vi "UHR-Fleezers Control (host) -Mau_stepping_gamma.vi"(0 "Tab Control":T5(tab)) -> ()   [LabVIEW 2013] (continued)
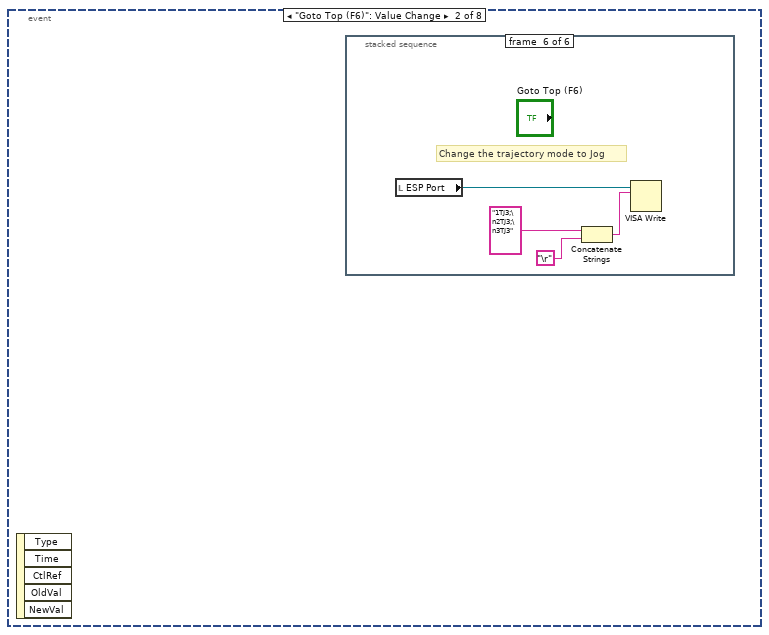
[diagram p4: hidden frame]
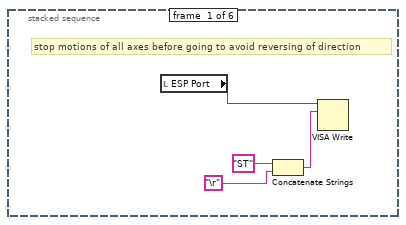
[diagram p5: hidden frame]
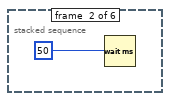
[diagram p6: hidden frame]
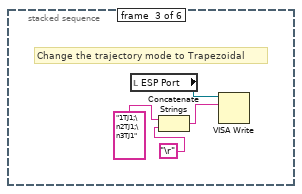
[diagram p7: hidden frame]
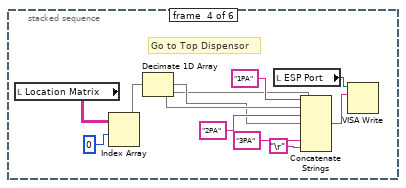
[diagram p8: hidden frame]
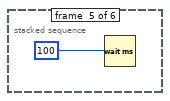
[diagram p9: hidden frame]
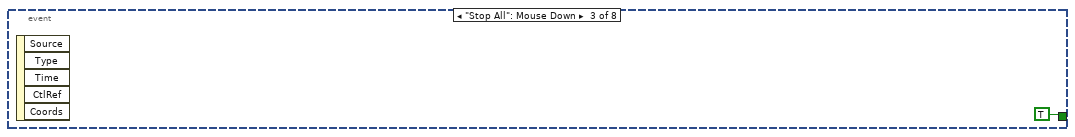
[diagram p10: hidden frame]
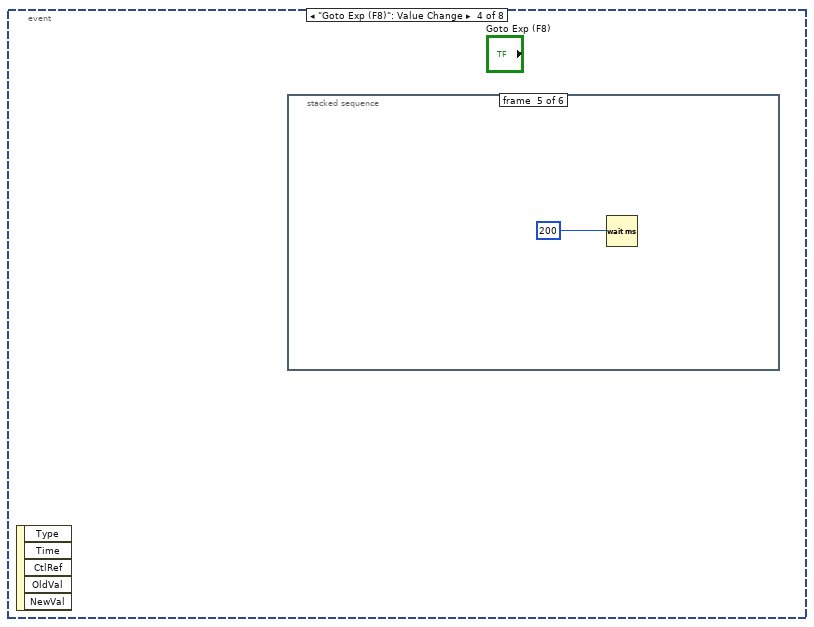
[diagram p11: hidden frame]
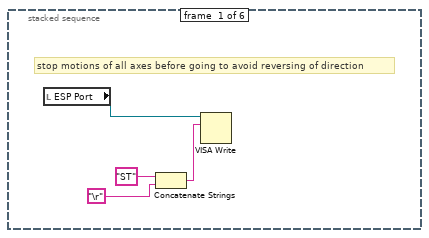
[diagram p12: hidden frame]
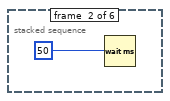
[diagram p13: hidden frame]
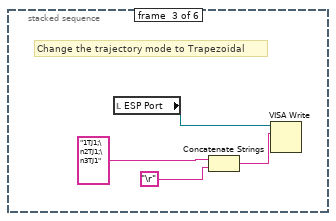
[diagram p14: hidden frame]
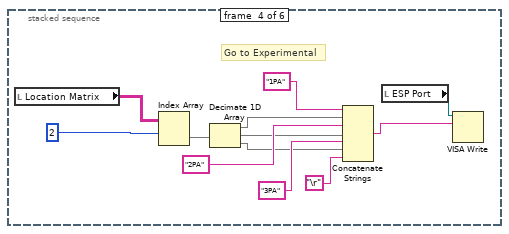
[diagram p15: hidden frame]
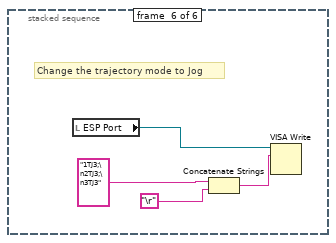
[diagram p16: hidden frame]
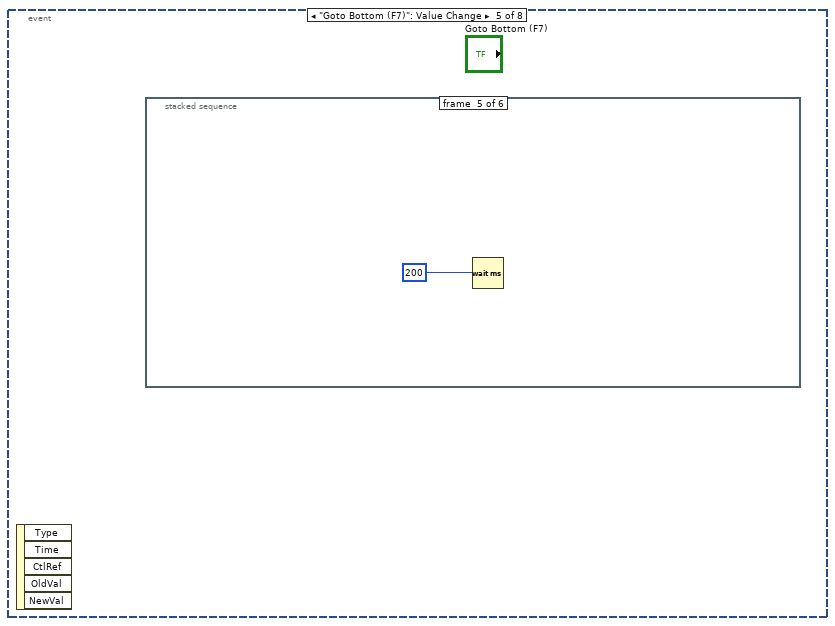
[diagram p17: hidden frame]
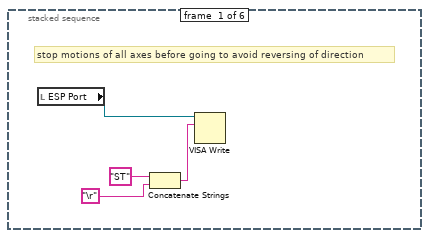
[diagram p18: hidden frame]
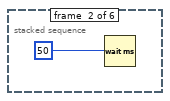
[diagram p19: hidden frame]
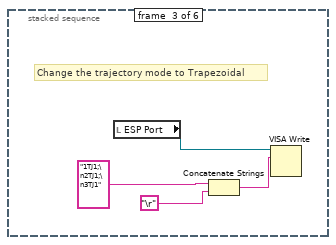
[diagram p20: hidden frame]
                n1984 = To Unsigned Long Integer(number=w3428) -> (unsigned 32bit integer=w3426:u32)
              }
            }
            n1985 = local read "Index"() -> (w3285:dbl)
            n1986 = call "Create new save file.vi"("Insert"="", "Ext"=".dat", "Index In"=w3285) -> ("Path Out"=w3244:path, "Index Out"=w3257:dbl)
            n1987 = local write "Save file name"(w3244) -> ()
            n1988 = local write "Index"(w3257) -> ()
            n1989 = local write "Save index"(w3257) -> ()
            n1990 = Array Size(array=w3268) -> (size(s)=w3269:i32)
            n1991 = Open/Create/Replace File(file path (use dialog)=w3244, operation (0:open)=T23."create", access (0:read/write)=enum16{"read/write", "read-only", "write-only"}."write-only") -> (refnum out=w3282:refnum<file>)  [unwired: 1 in, 4 out]
            n1992 = local write "Saving..."(TRUE ("Saving...")) -> ()
            n1993 = To Double Precision Float(number=w3269) -> (double precision float=w3267:dbl)
            n1994 = String Length(string="Comment (data description)") -> (length=w3265:i32)
            n1995 = To Double Precision Float(number=w3265) -> (double precision float=w3264:dbl)
            n1996 = Deny Access(7:w3282) -> (3:w3281:refnum<file>)  [unwired: 1 in, 2 out]
            n1997 = Build Array (concatenate)(w3267, w3268, w3264) -> (w3266:dbl[])
            n1998 = case "If fluorescence data to be saved" shown="True" w3255 {
              tunnel: w3244 -> [_ w3334]
              tunnel: [refnum<k0> refnum w3314] -> w3256
              frame False {
              }
              frame True {
                w3313 = 0.0
                n1999 = local read "APD Integration Time (s)"() -> (w3319:dbl)
                n2000 = local read "N APD Samp/step"() -> (w3312:dbl)
                n2001 = Path To String(path=w3334) -> (string=w3333:string)
                n2002 = String Length(string=w3333) -> (length=w3332:i32)
                n2003 = Subtract(x=w3332, y=4) -> (x-y=w3330:i32)
                n2004 = String Subset(string=w3333, length (rest)=w3330) -> (substring=w3329:string)  [unwired: 1 out]
                n2005 = Build Array(w3319, w3312, w3313, w3313, w3313, w3313, w3313, w3313) -> (w3316:dbl[])
                n2006 = Concatenate Strings(w3329, "_fl.dat" ("string")) -> (w3327:string)
                n2007 = Array Size(array=w3316) -> (size(s)=w3318:i32)
                n2008 = String To Path(string=w3327) -> (path=w3323:path)
                n2009 = Open/Create/Replace File(file path (use dialog)=w3323, operation (0:open)=T23."create", access (0:read/write)=enum16{"read/write", "read-only", "write-only"}."write-only") -> (refnum out=w3324:refnum<file>)  [unwired: 1 in, 4 out]
                n2010 = Deny Access(7:w3324) -> (3:w3320:refnum<file>)  [unwired: 1 in, 2 out]
                n2011 = To Double Precision Float(number=w3318) -> (double precision float=w3317:dbl)
                n2012 = Build Array (concatenate)(w3317, w3316) -> (w3315:dbl[])
                n2013 = Write to Binary File(file (use dialog)=w3320, data=w3315, 5:FALSE ("prepend array or string size? (T)"), 9:T29."big-endian, network order" ("byte order (0:big-endian, network order)")) -> (refnum out=w3314:refnum<file>)  [unwired: 1 in, 3 out]
              }
            }
            n2014 = case shown="True" w3242 {
              tunnel: w3244 -> [_ w3296]
              tunnel: [refnum<k0> refnum w3295] -> w3243
              frame False {
              }
              frame True {
                w3291 = 0.0 ("element")
                n2015 = Path To String(path=w3296) -> (string=w3310:string)
                n2016 = Build Array(w3291, w3291, w3291, w3291, w3291, w3291, w3291, w3291) -> (w3292:dbl[])
                n2017 = String Length(string=w3310) -> (length=w3309:i32)
                n2018 = Subtract(x=w3309, y=4) -> (x-y=w3307:i32)
                n2019 = Array Size(array=w3292) -> (size(s)=w3294:i32)
                n2020 = String Subset(string=w3310, length (rest)=w3307) -> (substring=w3306:string)  [unwired: 1 out]
                n2021 = To Double Precision Float(number=w3294) -> (double precision float=w3293:dbl)
                n2022 = Concatenate Strings(w3306, "_pos.dat" ("string")) -> (w3304:string)
                n2023 = Build Array (concatenate)(w3293, w3292) -> (w3290:dbl[])
                n2024 = String To Path(string=w3304) -> (path=w3300:path)
                n2025 = Open/Create/Replace File(file path (use dialog)=w3300, operation (0:open)=T23."create", access (0:read/write)=enum16{"read/write", "read-only", "write-only"}."write-only") -> (refnum out=w3301:refnum<file>)  [unwired: 1 in, 4 out]
                n2026 = Deny Access(7:w3301) -> (3:w3297:refnum<file>)  [unwired: 1 in, 2 out]
                n2027 = Write to Binary File(file (use dialog)=w3297, data=w3290, 5:FALSE ("prepend array or string size? (T)"), 9:T29."big-endian, network order" ("byte order (0:big-endian, network order)")) -> (refnum out=w3295:refnum<file>)  [unwired: 1 in, 3 out]
              }
            }
            n2028 = Write to Binary File(file (use dialog)=w3281, data=w3266, 5:w3262, 9:w3260) -> (refnum out=w3263:refnum<file>)  [unwired: 1 in, 3 out]
            n2029 = Write to Binary File(file (use dialog)=w3263, data="Comment (data description)", 5:w3262, 9:w3260) -> (refnum out=w3259:refnum<file>)  [unwired: 1 in, 3 out]
          }
        }
        n2030 = feedback-in #19(w3202) -> ()
        n2031 = feedback-in #20(w3229) -> ()
        n2032 = feedback-in #21(w3201) -> ()
        n2033 = feedback-in #22(w3212) -> ()
        n2034 = feedback-in #23(w3215) -> ()
        n2035 = feedback-in #24(w3228) -> ()
        n2036 = feedback-in #25(w3218) -> ()
      }
      frame #1 {
        n2037 = local read "Saving..."() -> (w3459:bool)
        n2038 = case shown="True" w3459 {
          tunnel: w3463 -> [_ w3473]
          tunnel: w3462 -> [_ w3487]
          tunnel: w3461 -> [_ w3483]
          tunnel: w3460 -> [_ w3482]
          tunnel: w3458 -> [_ w3481]
          tunnel: w3457 -> [_ w3476]
          tunnel: w3456 -> [_ w3475]
          tunnel: w3455 -> [_ w3474]
          tunnel: w3454 -> [_ w3472]
          tunnel: w3453 -> [_ w3470]
          tunnel: w3452 -> [_ w3469]
          tunnel: w3451 -> [_ w3468]
          tunnel: w3450 -> [_ w3467]
          tunnel: w3449 -> [_ w3466]
          tunnel: w3448 -> [_ w3465]
          tunnel: w3447 -> [_ w3464]
          frame False {
          }
          frame True {
            n2039 = Multiply(x=w3473, y=w3472) -> (x*y=→"Time (s)":dbl)
            n2040 = Less Or Equal?(x=w3473, y=w3481) -> (x <= y?=w3485:bool)
            n2041 = Or(x="Stop Saving", y="Abort save 2") -> (x .or. y?=w3477:bool)
            n2042 = Not(x=w3477) -> (.not. x?=w3486:bool)
            n2043 = And(x=w3485, y=w3486) -> (x .and. y?=w3484:bool)
            n2044 = case shown="True" w3484 {
              tunnel: w3487 -> [w3494 w3562]
              tunnel: [0.0 w3565] -> w3480
              tunnel: w3473 -> [_ w3563]
              tunnel: w3481 -> [_ w3564]
              tunnel: w3483 -> [_ w3559]
              tunnel: w3482 -> [_ _]
              tunnel: w3476 -> [w3492 w3552]
              tunnel: w3475 -> [w3491 w3553]
              tunnel: w3474 -> [_ w3551]
              tunnel: w3470 -> [_ w3550]
              tunnel: w3469 -> [_ w3504]
              tunnel: w3468 -> [_ w3543]
              tunnel: w3467 -> [_ w3521]
              tunnel: w3466 -> [w3489 w3502]
              tunnel: w3465 -> [w3490 w3501]
              tunnel: w3464 -> [_ w3498]
              frame False {
                w3488 = FALSE
                n2045 = Close File(refnum=w3494) -> ()  [unwired: 1 in, 2 out]
                n2046 = case shown="True" w3491 {
                  tunnel: w3492 -> [_ w3496]
                  frame False {
                  }
                  frame True {
                    n2047 = Close File(refnum=w3496) -> ()  [unwired: 1 in, 2 out]
                  }
                }
                n2048 = case shown="True" w3489 {
                  tunnel: w3490 -> [_ w3495]
                  frame False {
                  }
                  frame True {
                    n2049 = Close File(refnum=w3495) -> ()  [unwired: 1 in, 2 out]
                  }
                }
                n2050 = local write "Calibrating Trap..."(w3488) -> ()
                n2051 = call <vilib>:"Beep.vi"() -> ()  [unwired: 3 in, 9 out]
                n2052 = local write "Stop Saving"(w3488) -> ()
                n2053 = property on="Raster Scanning..." class="Bool (strict)"("Val(Sgnl)"=w3488) -> ()  [unwired: 2 in, 2 out]
                "Saving..." <- w3488
              }
              frame True {
                n2054 = local read "Calibrating Trap..."() -> (w3554:bool)
                n2055 = case "Write fl. data" shown="True" w3553 {
                  tunnel: w3552 -> [_ w3588]
                  tunnel: w3551 -> [_ w3587]
                  frame False {
                  }
                  frame True {
                    n2056 = Write to Binary File(file (use dialog)=w3588, data=w3587, 5:FALSE ("prepend array or string size? (T)"), 9:T29."big-endian, network order" ("byte order (0:big-endian, network order)")) -> ()  [unwired: 1 in, 4 out]
                  }
                }
                n2057 = Greater?(x="Save ave N", y=1.0) -> (0:w3557:bool)
                n2058 = Not(x=w3554) -> (.not. x?=w3556:bool)
                n2059 = And(x=w3556, y=w3557) -> (x .and. y?=w3499:bool)
                n2060 = case shown="True" w3499 {
                  tunnel: w3498 -> [w3568 w3579]
                  tunnel: [w3568 w3571] -> w3497
                  tunnel: "Save ave N" -> [_ w3572]
                  frame False {
                  }
                  frame True {
                    w3569 = 2 ("dimension size")
                    n2061 = Array Size(array=w3579) -> (size(s)=w3573:i32)
                    n2062 = Divide(x=w3573, y=w3569) -> (x/y=w3577:dbl)
                    n2063 = Reshape Array(w3579, w3577, w3569) -> (w3578:u64[][])
                    n2064 = Transpose 2D Array(2D array=w3578) -> (transposed array=w3576:u64[][])
                    n2065 = for {
                      tunnel: w3576 -> [w3581] mode=indexing
                      tunnel: [w3580] -> w3570 mode=indexing
                      tunnel: w3572 -> [w3582]
                      workers-P: _ -> [_]
                      n2066 = call "downsample 1D array - U64.vi"("Ave N"=w3582, "Array In"=w3581) -> ("Array Out"=w3580:u64[])  [unwired: 1 in]
                    }
                    n2067 = Transpose 2D Array(2D array=w3570) -> (transposed array=w3575:u64[][])
                    n2068 = Divide(x=w3573, y=w3572) -> (x/y=w3574:dbl)
                    n2069 = Reshape Array(w3575, w3574) -> (w3571:u64[])
                  }
                }
                n2070 = case shown="True" w3499 {
                  tunnel: w3559 -> [w3591 w3603]
                  tunnel: [w3591 w3595] -> w3555
                  tunnel: "Save ave N" -> [_ w3596]
                  tunnel: w3550 -> [_ w3594]
                  frame False {
                    # "don't downsample data for trap calibration"
                  }
                  frame True {
                    n2071 = Array Size(array=w3603) -> (size(s)=w3597:i32)
                    n2072 = Array Size(array=w3594) -> (size(s)=w3593:i32)
                    n2073 = Divide(x=w3597, y=w3593) -> (x/y=w3601:dbl)
                    n2074 = Reshape Array(w3603, w3601, w3593) -> (w3602:i16[][])
                    n2075 = Transpose 2D Array(2D array=w3602) -> (transposed array=w3600:i16[][])
                    n2076 = for {
                      tunnel: w3600 -> [w3606] mode=indexing
                      tunnel: [w3605] -> w3592 mode=indexing
                      tunnel: w3596 -> [w3604]
                      workers-P: _ -> [_]
                      n2077 = call "downsample 1D array - I16.vi"("Ave N"=w3604, "Array In"=w3606) -> ("Array Out"=w3605:i16[])  [unwired: 1 out]
                    }
                    n2078 = Transpose 2D Array(2D array=w3592) -> (transposed array=w3599:i16[][])
                    n2079 = Divide(x=w3597, y=w3596) -> (x/y=w3598:dbl)
                    n2080 = Reshape Array(w3599, w3598) -> (w3595:i16[])
                  }
                }
                n2081 = Index Array(array=w3521, index=1) -> (element=w3524:waveform(dbl))
                n2082 = Index Array(array=w3521, index=0) -> (element=w3526:waveform(dbl))
                n2083 = Unbundle By Name(w3524) -> ("Y"=w3528:dbl[])
                n2084 = Unbundle By Name(w3526) -> ("Y"=w3536:dbl[])
                n2085 = case "Write trap pos. data" shown="True" w3502 {
                  tunnel: w3501 -> [_ w3584]
                  tunnel: w3497 -> [_ w3583]
                  frame False {
                  }
                  frame True {
                    n2086 = Write to Binary File(file (use dialog)=w3584, data=w3583, 5:FALSE ("prepend array or string size? (T)"), 9:T29."big-endian, network order" ("byte order (0:big-endian, network order)")) -> ()  [unwired: 1 in, 4 out]
                  }
                }
                n2087 = Write to Binary File(file (use dialog)=w3562, data=w3555, 5:FALSE ("prepend array or string size? (T)"), 9:T29."big-endian, network order" ("byte order (0:big-endian, network order)")) -> ()  [unwired: 1 in, 4 out]
                n2088 = feedback #26(w3528) -> (w3530:dbl[])
                n2089 = Build Array (concatenate)(w3530, w3528) -> (w3529:dbl[])
                n2090 = Select(t=w3528, s=w3504, f=w3529) -> (s? t:f=w3514:dbl[])
                n2091 = feedback-in #26(w3514) -> ()
                n2092 = feedback #27(w3536) -> (w3549:dbl[])
                n2093 = Build Array (concatenate)(w3549, w3536) -> (w3548:dbl[])
                n2094 = Select(t=w3536, s=w3504, f=w3548) -> (s? t:f=w3523:dbl[])
                n2095 = feedback-in #27(w3523) -> ()
                n2096 = Divide(x=w3563, y=w3564) -> (x/y=w3566:dbl)
                n2097 = Multiply(x=w3566, y=100.0) -> (x*y=w3565:dbl)
                n2098 = Build Array(w3523, w3514) -> (→"Saved APD":dbl[][])
                n2099 = Array Size(array=w3523) -> (size(s)=w3541:i32)
                n2100 = Unbundle By Name(w3543) -> ("Y"=w3547:dbl[])
                n2101 = Subtract(x=w3541, y="N pts to average") -> (x-y=w3517:i32)
                n2102 = Multiply(x="N pts to average", y=u16 2) -> (x*y=w3518:u16)
                n2103 = Subtract(x=w3541, y=w3518) -> (x-y=w3516:i32)
                n2104 = feedback #28(w3547) -> (w3546:dbl[])
                n2105 = Build Array (concatenate)(w3546, w3547) -> (w3545:dbl[])
                n2106 = Select(t=w3547, s=w3504, f=w3545) -> (s? t:f=w3544:dbl[])
                "Trap Delta Graph" <- w3544
                n2107 = feedback-in #28(w3544) -> ()
                n2108 = Array Subset(array=w3523, index=w3517, length="N pts to average") -> (w3540:dbl[])
                n2109 = Array Subset(array=w3523, index=w3516, length="N pts to average") -> (w3539:dbl[])
                n2110 = Array Subset(array=w3514, index=w3517, length="N pts to average") -> (w3520:dbl[])
                n2111 = Array Subset(array=w3514, index=w3516, length="N pts to average") -> (w3519:dbl[])
                n2112 = call-poly <vilib>:"Mean.vi"("X"=w3540) -> ("mean"=w3538:dbl)  [unwired: 1 out]
                n2113 = call-poly <vilib>:"Mean.vi"("X"=w3520) -> ("mean"=w3513:dbl)  [unwired: 1 out]
                n2114 = call-poly <vilib>:"Mean.vi"("X"=w3539) -> ("mean"=w3537:dbl)  [unwired: 1 out]
                n2115 = call-poly <vilib>:"Mean.vi"("X"=w3519) -> ("mean"=w3512:dbl)  [unwired: 1 out]
                n2116 = Subtract(x=w3513, y=w3512) -> (x-y=w3503:dbl)
                "Delta Fl. 2" <- w3503
                n2117 = Subtract(x=w3538, y=w3537) -> (x-y=w3535:dbl)
                "Delta Fl. 1" <- w3535
                n2118 = Initialize Array(w3535, 1 ("dimension size")) -> (w3532:dbl[])
                n2119 = Initialize Array(w3503, 1 ("dimension size")) -> (w3509:dbl[])
                n2120 = feedback #29(w3532) -> (w3533:dbl[])
                n2121 = Build Array (concatenate)(w3533, w3532) -> (w3531:dbl[])
                n2122 = feedback #30(w3509) -> (w3510:dbl[])
                n2123 = Build Array (concatenate)(w3510, w3509) -> (w3508:dbl[])
                n2124 = Select(t=w3532, s=w3504, f=w3531) -> (s? t:f=w3507:dbl[])
                n2125 = feedback-in #29(w3507) -> ()
                n2126 = Select(t=w3509, s=w3504, f=w3508) -> (s? t:f=w3506:dbl[])
                n2127 = feedback-in #30(w3506) -> ()
                n2128 = Build Array(w3507, w3506) -> (→"Save APD Deriv":dbl[][])
              }
            }
            "Progress" <- w3480
            "Progress 2" <- w3480
          }
        }
      }
    }
    n2129 = Bundle By Name(cluster=w2224, "Green FB Ch 0"=w2223, "Green FB Ch 1"=w2222) -> (w2202:T48)
    "Green FB Signals (V)" <- w2202
    n2130 = Unbundle By Name(w2202) -> ("Green FB Ch 2"=→"Green FB Plot":dbl)
    n2131 = local read "wait to reset values"() -> (w2294:bool)
    n2132 = Not(x=w2291) -> (.not. x?=w2295:bool)
    n2133 = And(x=w2295, y=w2294) -> (x .and. y?=w2296:bool)
    n2134 = case "Part of MCL raster scanning: returns to initial positions after scan done" shown="False" w2296 {
      tunnel: w2299 -> [w3032 w3039]
      tunnel: [w3032 w3038] -> w2298
      tunnel: w2293 -> [w3031 w3037]
      tunnel: [w3031 w3036] -> w2292
      frame False {
      }
      frame True {
        w3047 = 10.0 ("y")
        w3046 = 32767.0 ("y")
        # "to return scan values\nafter a synchronous \nAOM scan"
        n2135 = local read "AO2"() -> (w3040:dbl)
        n2136 = local read "AO1"() -> (w3041:dbl)
        n2137 = local write "wait to reset values"(FALSE ("wait to reset values")) -> ()
        n2138 = Multiply(x=w3041, y=w3046) -> (x*y=w3043:dbl)
        n2139 = Multiply(x=w3040, y=w3046) -> (x*y=w3045:dbl)
        n2140 = Divide(x=w3043, y=w3047) -> (x/y=w3042:dbl)
        n2141 = Divide(x=w3045, y=w3047) -> (x/y=w3044:dbl)
        n2142 = To Word Integer(number=w3042) -> (16bit integer=w3048:i16)
        n2143 = To Word Integer(number=w3044) -> (16bit integer=w3049:i16)
        n2144 = local read "Total Counts (ticks)"() -> (w3033:u32)
        n2145 = xnode "Read/Write Control"("FPGA VI Reference In"=w3039, "error in"=w3037, "AO1"=w3048, "AO2"=w3049, "MCL count"=w3033) -> ("FPGA VI Reference Out"=w3038:T19, "error out"=w3036:errorcluster)
        n2146 = local read "Scan Range (V)\n(of steps)"() -> (w3034:dbl)
        n2147 = property on="Scan Range (V)\n(of steps)" class="DigNum (strict)"("Val(Sgnl)"=w3034) -> ()  [unwired: 2 in, 2 out]
      }
    }
    n2148 = node-c288() -> ()  [unwired: 2 out]
  }
  n2149 = node-c288(3 ("Processor")) -> (w74:T24)  [unwired: 3 out]
  n2150 = timed-loop "Oscillate AOD (debugging)" {
    tunnel: w24 -> [w3608]
    tunnel: [w3607] -> w36
    timing: w74 -> [_]
    timing-out: [_] -> w73
    stop <- w3607 stop-if-true
    n2151 = node-c288() -> ()  [unwired: 2 out]
    n2152 = event shown="[0] \"Oscillate Set 2\", \"Fish for Tether\": Value Change" {
      selector: _ -> [_ _ _]
      dyn-events: _ -> [_ _ _]
      timeout: _ -> [_ _ _]
      tunnel: w3608 -> [w3615 _ _]
      tunnel: [FALSE ("Stop All") _ w3890] -> w3607
      event "Oscillate Set 2", "Fish for Tether": Value Change {
        n2153 = event-data() -> ()  [unwired: 6 out]
        n2154 = local read "Oscillate Set 2"() -> (w3614:bool)
        n2155 = Or(x=w3614, y="Fish for Tether") -> (x .or. y?=w3612:bool)
        n2156 = case shown="True" w3612 {
          tunnel: w3615 -> [_ w3618]
          tunnel: "Fish for Tether" -> [_ w3617]
          frame False {
          }
          frame True {
            n2157 = case shown="True" w3617 {
              frame False {
              }
              frame True {
                n2158 = local write "Scan axis 2"(TRUE) -> ()
                n2159 = local write "Tether"(FALSE ("Tether")) -> ()
              }
            }
            n2160 = node-c288("Period") -> (w3620:T24)  [unwired: 3 out]
            n2161 = timed-loop "Oscillate AOD" {
              timing: w3620 -> [_]
              timing-out: [_] -> w3619
              tunnel: w3618 -> [w3630]
              tunnel: w3617 -> [w3629]
              i -> [w3632]
              stop <- w3628 stop-if-true
              n2162 = node-c288() -> (w3631:i64)  [unwired: 1 out]
              n2163 = flat-sequence {
                tunnel: w3632 -> [w3658]
                tunnel: w3631 -> [w3657]
                tunnel: w3630 -> [w3641]
                tunnel: w3629 -> [w3643]
                tunnel: [w3643] -> w3627
                tunnel: [w3642] -> w3626
                tunnel: [w3640] -> w3625
                tunnel: [w3637] -> w3623
                tunnel: w3627 -> [w3701]
                tunnel: w3626 -> [w3699]
                tunnel: w3625 -> [w3698]
                tunnel: [w3697] -> w3624
                tunnel: w3623 -> [w3696]
                tunnel: [w3765] -> w3628
                tunnel: w3624 -> [w3763]
                frame #0 {
                  n2164 = Divide(x=w3657, y=i64 1000) -> (x/y=w3652:dbl)
                  n2165 = Multiply(x=w3652, y=w3658) -> (x*y=w3654:dbl)
                  n2166 = Multiply(x="Osc. freq. (Hz)", y=6.283185307179586) -> (x*y=w3655:dbl)
                  n2167 = Multiply(x=w3655, y=w3654) -> (x*y=w3639:dbl)
                  n2168 = local read "BD 1 Frequency 2 (MHz)"() -> (w3636:dbl)
                  n2169 = local read "BD 1 Frequency 1 (MHz)"() -> (w3633:dbl)
                  n2170 = case shown="True" w3643 {
                    tunnel: w3639 -> [w3664 w3679]
                    tunnel: w3636 -> [_ w3689]
                    tunnel: [w3661 w3673] -> w3644
                    tunnel: [FALSE w3682] -> w3640
                    tunnel: [0.0 w3675] -> w3637
                    tunnel: w3633 -> [_ w3674]
                    frame False {
                      n2171 = Sine(x=w3664) -> (sin(x)=w3662:dbl)
                      n2172 = Multiply(x=w3662, y="Osc. amp. (MHz)") -> (x*y=w3661:dbl)
                    }
                    frame True {
                      n2173 = Cosine(x=w3679) -> (cos(x)=w3672:dbl)
                      n2174 = Subtract(x=w3689, y=w3674) -> (x-y=w3688:dbl)
                      n2175 = Equal?(x=-1, y=w3672) -> (x = y?=w3670:bool)
                      n2176 = Decrement(x=w3672) -> (x-1=w3691:dbl)
                      n2177 = Subtract(x=w3688, y="Closest Delta (MHz)") -> (x-y=w3685:dbl)
                      n2178 = Select(t="Pause at Closest Delta (s)", s=w3670, f=0) -> (s? t:f=w3668:dbl)
                      n2179 = Divide(x=w3691, y=2.0) -> (x/y=w3686:dbl)
                      n2180 = Multiply(x=1000, y=w3668) -> (x*y=w3666:dbl)
                      n2181 = Multiply(x=w3686, y=w3685) -> (x*y=w3673:dbl)
                      n2182 = local read "Vec Mean of T1 T2"() -> (w3681:dbl[])
                      n2183 = Wait (ms)(milliseconds to wait=w3666) -> ()  [unwired: 1 out]
                      n2184 = Greater?(x=w3681, y="Stop F (pN)") -> (0:w3683:bool[])
                      n2185 = Or Array Elements(Boolean array=w3683) -> (logical OR=w3682:bool)
                      n2186 = Divide(x=w3679, y=6.283185307179586) -> (x/y=w3678:dbl)
                      n2187 = Round Toward +Infinity(x=w3678) -> (ceil(x): smallest int >= x=w3675:dbl)
                      "Attempts" <- w3675
                      n2188 = Greater?(x=w3675, y="Attempt Limit") -> (0:w3677:bool)
                      n2189 = case shown="True" w3677 {
                        frame False {
                        }
                        frame True {
                          n2190 = local write "Fish for Tether"(FALSE ("Fish for Tether")) -> ()
                          n2191 = call <vilib>:"Beep.vi"() -> ()  [unwired: 3 in, 9 out]
                          n2192 = local read "Messages"() -> (w3693:string)
                          n2193 = call "Update messages.vi"("Message to add"="Tether fishing timeout." ("Messages"), "Old message string"=w3693) -> ("New message string"=→"Messages":string)
                        }
                      }
                    }
                  }
                  n2194 = local read "Y RF Frequency Limits (MHz)"() -> (w3645:T16)
                  n2195 = local read "X RF Frequency Limits (MHz)"() -> (w3646:T16)
                  n2196 = local read "BD 1 Frequency 3 (MHz)"() -> (w3651:dbl)
                  n2197 = local read "BD 2 Frequency 2 (MHz)"() -> (w3635:dbl)
                  n2198 = Select(t=w3636, s="Scan axis 2", f=w3635) -> (s? t:f=w3647:dbl)
                  n2199 = Add(x=w3644, y=w3647) -> (x+y=w3642:dbl)
                  n2200 = Select(t=w3642, s="Scan axis 2", f=w3636) -> (s? t:f=w3634:dbl)
                  n2201 = Select(t=w3635, s="Scan axis 2", f=w3642) -> (s? t:f=w3649:dbl)
                  n2202 = local read "BD 2 Frequency 3 (MHz)"() -> (w3650:dbl)
                  n2203 = call "set RF board frequency - interlace.vi"("Board 2 Frequency Limits"=w3645, "Board 1 Frequency Limits"=w3646, "FPGA VI Reference In"=w3641, "Board 2 Frequency 3 (MHz)"=w3650, "Board 1 Frequency 3 (MHz)"=w3651, "Board 2 Frequency 2 (MHz)"=w3635, "Board 2 Frequency 1 (MHz)"=w3649, "Board 1 Frequency 2 (MHz)"=w3634, "Board 1 Frequency 1  (MHz)"=w3633) -> ()  [unwired: 1 in, 2 out]
                }
                frame #1 {
                  n2204 = And(x=w3701, y=w3698) -> (x .and. y?=w3700:bool)
                  n2205 = case "Only if were fishing and now formed tether" shown="True" w3700 {
                    tunnel: w3699 -> [w3703 w3715]
                    tunnel: [w3702 w3714] -> w3697
                    tunnel: w3696 -> [_ w3710]
                    frame False {
                      n2206 = local read "Fish for Tether"() -> (w3702:bool)
                      n2207 = case shown="True" w3702 {
                        tunnel: w3703 -> [_ _]
                        frame False {
                        }
                        frame True {
                        }
                      }
                    }
                    frame True {
                      w3714 = FALSE ("Fish for Tether")
                      n2208 = call <vilib>:"Beep.vi"() -> ()  [unwired: 3 in, 9 out]
                      n2209 = Number To Decimal String(number=w3710, width (-)=i16 1) -> (decimal integer string=w3708:string)
                      n2210 = case shown="\"2\", \"3\", \"4\", \"5\", \"6\"" "Then..." {
                        selector: "Then..." -> [_ w3718]
                        tunnel: w3715 -> [w3717 _]
                        frame "1", Default {
                          # "do nothing"
                          n2211 = property on="BD 1 Frequency 1 (MHz)" class="DigNum (strict)"("Val(Sgnl)"=w3717) -> ()  [unwired: 2 in, 2 out]
                        }
                        frame "2", "3", "4", "5", "6" {
                          n2212 = flat-sequence {
                            tunnel: w3718 -> [w3720]
                            frame #0 {
                              n2213 = property on="Trap Delta (MHz)" class="DigNum (strict)"("Val(Sgnl)"="Move to Delta 1 (MHz)") -> ()  [unwired: 2 in, 2 out]
                            }
                            frame #1 {
                              n2214 = case shown="\"5\", \"6\"" w3720 {
                                selector: w3720 -> [w3723 w3733 _]
                                frame "3", "4" {
                                n2215 = flat-sequence {
                                tunnel: w3723 -> [w3724]
                                tunnel: [w3724] -> w3721
                                tunnel: [w3726] -> w3722
                                tunnel: w3721 -> [w3726]
                                tunnel: w3722 -> [w3730]
                                frame #0 {
                                n2216 = property on="Green Laser ON/Interlacing" class="Bool (strict)"("Val(Sgnl)"=TRUE ("Value (Signaling)")) -> ()  [unwired: 2 in, 2 out]
                                }
                                frame #1 {
                                n2217 = Multiply(x="Wait Before Save (s)", y=u32 1000 ("x")) -> (x*y=w3728:u32)
                                n2218 = Wait (ms)(milliseconds to wait=w3728) -> ()  [unwired: 1 out]
                                }
                                frame #2 {
                                n2219 = property on="Start Saving" class="Bool (strict)"("Value"=TRUE ("Start Saving")) -> ()  [unwired: 2 in, 2 out]
                                n2220 = case shown="Default" w3730 {
                                frame Default {
                                }
                                frame "4" {
                                n2221 = property on="Fl. Triggered..." class="Bool (strict)"("Val(Sgnl)"=TRUE ("Value (Signaling)")) -> ()  [unwired: 2 in, 2 out]
                                }
                                }
                                }
                                }
                                }
                                frame "5", "6" {
                                n2222 = stacked-sequence {
                                tunnel: w3733 -> [_ _ _ _ _ _ _ _ w3750 _ _]
                                frame #0 {
                                n2223 = Replace Array Subset(array=u32[] [0] ("Index Values"), new element="Raster Set Upon Tether", index=0) -> (w3734:u32[])
                                n2224 = property on="Saved AOD Raster Scan Parameter Sets" class="Arr (strict)"("Index Values"=w3734) -> ()  [unwired: 2 in, 2 out]
                                }
                                frame #1 {
                                n2225 = Wait (ms)(milliseconds to wait=u32 500) -> ()  [unwired: 1 out]
                                }
                                frame #2 {
                                n2226 = property on="Load parameters" class="Bool (strict)"("Val(Sgnl)"=TRUE ("Value (Signaling)")) -> ()  [unwired: 2 in, 2 out]
                                }
                                frame #3 {
                                n2227 = Wait (ms)(milliseconds to wait=u32 500) -> ()  [unwired: 1 out]
                                }
                                frame #4 {
                                n2228 = property on="Trap Raster Scan" class="Bool (strict)"("Val(Sgnl)"=TRUE ("Value (Signaling)")) -> ()  [unwired: 2 in, 2 out]
                                }
                                frame #5 {
                                n2229 = Wait (ms)(milliseconds to wait=u32 2000) -> ()  [unwired: 1 out]
                                }
                                frame #6 {
                                n2230 = while {
                                stop <- w3745 stop-if-true
                                n2231 = local read "Raster Scanning..."() -> (w3744:bool)
                                n2232 = local read "Saving..."() -> (w3747:bool)
                                n2233 = Wait (ms)(milliseconds to wait=u32 100) -> ()  [unwired: 1 out]
                                n2234 = Not(x=w3747) -> (.not. x?=w3746:bool)
                                n2235 = Not(x=w3744) -> (.not. x?=w3743:bool)
                                n2236 = And(x=w3746, y=w3743) -> (x .and. y?=w3745:bool)
                                }
                                }
                                frame #7 {
                                n2237 = property on="Trap Delta (MHz)" class="DigNum (strict)"("Val(Sgnl)"="Move to Delta 2 (MHz)") -> ()  [unwired: 2 in, 2 out]
                                }
                                frame #8 {
                                n2238 = local read "Tether"() -> (w3751:bool)
                                n2239 = case shown="True" w3751 {
                                tunnel: w3750 -> [_ w3752]
                                frame False {
                                }
                                frame True {
                                n2240 = flat-sequence {
                                tunnel: w3752 -> [w3754]
                                frame #0 {
                                n2241 = Wait (ms)(milliseconds to wait=u32 500) -> ()  [unwired: 1 out]
                                }
                                frame #1 {
                                n2242 = case shown="\"6\"" w3754 {
                                frame Default {
                                }
                                frame "6" {
                                n2243 = property on="Green Laser ON/Interlacing" class="Bool (strict)"("Val(Sgnl)"=TRUE ("Green Laser ON/Interlacing")) -> ()  [unwired: 2 in, 2 out]
                                }
                                }
                                }
                                frame #2 {
                                n2244 = Wait (ms)(milliseconds to wait=u32 500) -> ()  [unwired: 1 out]
                                }
                                frame #3 {
                                n2245 = local write "Start Saving"("Save at end (5, 6)") -> ()
                                }
                                }
                                }
                                }
                                }
                                frame #9 {
                                n2246 = local read "Bead Sep. Int. Time (s)"() -> (w3760:dbl)
                                n2247 = Multiply(x=w3760, y=1000.0) -> (x*y=w3759:dbl)
                                n2248 = Wait (ms)(milliseconds to wait=w3759) -> ()  [unwired: 1 out]
                                }
                                frame #10 {
                                n2249 = property on="Rescale on Mean" class="Bool (strict)"("Val(Sgnl)"=TRUE ("Value (Signaling)")) -> ()  [unwired: 2 in, 2 out]
                                }
                                }
                                }
                                frame "2", Default {
                                }
                              }
                            }
                          }
                        }
                      }
                      n2250 = Concatenate Strings("Formed tether in ", w3708, " attempt(s)." ("string")) -> (w3705:string)
                      n2251 = local read "Messages"() -> (w3712:string)
                      n2252 = local write "Fish for Tether"(w3714) -> ()
                      n2253 = call "Update messages.vi"("Message to add"=w3705, "Old message string"=w3712) -> ("New message string"=w3711:string)
                      n2254 = local write "Messages"(w3711) -> ()
                      n2255 = Get Date/Time In Seconds() -> (seconds since 1Jan1904=→"Time tether formed":timestamp)
                      "Tether" <- "Tether Alarm?"
                    }
                  }
                }
                frame #2 {
                  n2256 = local read "Oscillate Set 2"() -> (w3764:bool)
                  n2257 = local read "Stop All"() -> (w3766:bool)
                  n2258 = Not Or(1:w3763, 2:w3764) -> (0:w3762:bool)
                  n2259 = Compound Arithmetic op=OR(w3766, w3762) -> (w3765:bool)
                }
              }
              n2260 = node-c288() -> ()  [unwired: 2 out]
            }
            n2261 = node-c288(w3619) -> ()  [unwired: 1 out]
          }
        }
      }
      event "Fl. Triggered...": Value Change {
        n2262 = event-data() -> ()  [unwired: 7 out]
        n2263 = case shown="True" "Fl. Triggered..." {
          frame False {
          }
          frame True {
            n2264 = node-c288() -> (w3778:T24)  [unwired: 4 out]
            n2265 = timed-loop {
              timing: w3778 -> [_]
              timing-out: [_] -> w3777
              tunnel: "Action" -> [w3782]
              shift-right: [w3779] -> _
              shift-left: u8 255 -> [w3781]
              stop <- w3783 stop-if-true
              n2266 = node-c288() -> ()  [unwired: 2 out]
              n2267 = flat-sequence {
                tunnel: w3782 -> [w3795]
                tunnel: w3781 -> [w3792]
                tunnel: [w3791] -> w3780
                tunnel: [w3881] -> w3783
                tunnel: w3780 -> [w3880]
                tunnel: [w3880] -> w3779
                frame #0 {
                  n2268 = local read "Delta Fl. 2"() -> (w3786:dbl)
                  n2269 = local read "Delta Fl. 1"() -> (w3787:dbl)
                  n2270 = Select(t=w3787, s="APD to Watch", f=w3786) -> (s? t:f=w3785:dbl)
                  n2271 = Multiply(x="Fl. Delta Thresh. (kHz)", y=1000.0) -> (x*y=w3794:dbl)
                  n2272 = Greater?(x=w3785, y=w3794) -> (0:w3789:bool)
                  n2273 = Or(x="Force Yank", y=w3789) -> (x .or. y?=w3790:bool)
                  n2274 = case shown="True" w3790 {
                    tunnel: w3795 -> [_ w3805]
                    tunnel: w3792 -> [w3797 w3801]
                    tunnel: [w3797 w3798] -> w3791
                    frame False {
                    }
                    frame True {
                      n2275 = flat-sequence {
                        tunnel: w3802 -> [w3811]
                        tunnel: [w3811] -> w3806
                        tunnel: w3805 -> [w3810]
                        tunnel: [w3810] -> w3804
                        tunnel: [w3809] -> w3803
                        tunnel: w3801 -> [w3808]
                        tunnel: [w3807] -> w3800
                        tunnel: w3806 -> [w3836]
                        tunnel: w3804 -> [w3835]
                        tunnel: w3803 -> [w3834]
                        tunnel: w3800 -> [w3833]
                        tunnel: [w3833] -> w3799
                        tunnel: w3799 -> [w3878]
                        tunnel: [w3878] -> w3798
                        frame #0 {
                          n2276 = call <vilib>:"Beep.vi"() -> ()  [unwired: 3 in, 9 out]
                          n2277 = local write "Waiting"(FALSE ("Waiting")) -> ()
                          n2278 = Increment(x=w3808) -> (x+1=w3807:u8)
                          n2279 = case shown="\"Yank\"" w3810 {
                            tunnel: w3807 -> [_ _ w3817]
                            frame "Image" {
                              n2280 = property on="Confocal Image" class="Bool (strict)"("Val(Sgnl)"=TRUE ("Value (Signaling)")) -> ()  [unwired: 2 in, 2 out]
                            }
                            frame "Alarm", Default {
                            }
                            frame "Yank" {
                              n2281 = flat-sequence {
                                tunnel: w3817 -> [w3820]
                                tunnel: [w3819] -> w3816
                                tunnel: ["N Array El"] -> w3815
                                tunnel: w3816 -> [w3830]
                                tunnel: w3815 -> [w3826]
                                frame #0 {
                                n2282 = Multiply(x="Yank Delay (s)", y=1000.0) -> (x*y=w3823:dbl)
                                n2283 = Quotient & Remainder(x=w3820, y="N Array El") -> (x-y*floor(x/y)=w3819:u8)  [unwired: 1 out]
                                n2284 = Wait (ms)(milliseconds to wait=w3823) -> ()  [unwired: 1 out]
                                }
                                frame #1 {
                                n2285 = Random Number (0-1)() -> (number: 0 to 1=w3827:dbl)
                                n2286 = Multiply(x=w3826, y=w3827) -> (x*y=w3825:dbl)
                                n2287 = Round Toward -Infinity(1:w3825) -> (0:w3824:dbl)
                                n2288 = Select(t=w3824, s="Random Choice", f=w3830) -> (s? t:f=w3828:dbl)
                                n2289 = Index Array(array="Yank to Delta Array (MHz)", index=w3828) -> (element=w3831:dbl)
                                n2290 = property on="Trap Delta (MHz)" class="DigNum (strict)"("Val(Sgnl)"=w3831) -> ()  [unwired: 2 in, 2 out]
                                }
                              }
                            }
                          }
                          n2291 = local read "Time (s)"() -> (w3809:dbl)
                          "Fl. High" <- TRUE ("Yanking")
                        }
                        frame #1 {
                          n2292 = node-c288() -> (w3838:T24)  [unwired: 4 out]
                          n2293 = timed-loop {
                            timing: w3838 -> [_]
                            timing-out: [_] -> w3837
                            tunnel: w3836 -> [w3854]
                            tunnel: w3835 -> [w3852]
                            tunnel: w3834 -> [w3851]
                            stop <- w3853 stop-if-true
                            n2294 = node-c288() -> ()  [unwired: 2 out]
                            n2295 = local read "Fl. Delta Thresh. (kHz)"() -> (w3846:dbl)
                            n2296 = local read "Fl. Triggered..."() -> (w3855:bool)
                            n2297 = local read "Delta Fl. 1"() -> (w3842:dbl)
                            n2298 = local read "Delta Fl. 2"() -> (w3840:dbl)
                            n2299 = local read "Stop All"() -> (w3849:bool)
                            n2300 = local read "APD to Watch"() -> (w3841:bool)
                            n2301 = Select(t=w3842, s=w3841, f=w3840) -> (s? t:f=w3839:dbl)
                            n2302 = Not(x=w3855) -> (.not. x?=w3850:bool)
                            n2303 = Multiply(x=w3846, y=1000.0) -> (x*y=w3845:dbl)
                            n2304 = Negate(x=w3845) -> (-x=w3844:dbl)
                            n2305 = Less?(x=w3839, y=w3844) -> (x < y?=w3848:bool)
                            n2306 = Compound Arithmetic op=OR(w3848, w3849, w3850, "Force Reset") -> (w3853:bool)
                            n2307 = case shown="True" w3853 {
                              tunnel: w3854 -> [_ w3866]
                              tunnel: w3852 -> [_ w3865]
                              tunnel: w3851 -> [_ w3863]
                              frame False {
                              }
                              frame True {
                                n2308 = case shown="\"Yank\"" w3865 {
                                tunnel: w3866 -> [_ w3867]
                                frame "Image", Default {
                                }
                                frame "Yank" {
                                n2309 = flat-sequence {
                                tunnel: [w3872] -> w3868
                                tunnel: w3867 -> [w3872]
                                tunnel: w3868 -> [w3873]
                                frame #0 {
                                n2310 = local read "Yank Delay (s)"() -> (w3871:dbl)
                                n2311 = Multiply(x=w3871, y=1000.0) -> (x*y=w3869:dbl)
                                n2312 = Wait (ms)(milliseconds to wait=w3869) -> ()  [unwired: 1 out]
                                }
                                frame #1 {
                                n2313 = property on="Trap Delta (MHz)" class="DigNum (strict)"("Val(Sgnl)"=w3873) -> ()  [unwired: 2 in, 2 out]
                                }
                                }
                                }
                                }
                                n2314 = local read "Time (s)"() -> (w3864:dbl)
                                n2315 = Subtract(x=w3864, y=w3863) -> (x-y=w3860:dbl)
                                "Duration (s)" <- w3860
                                n2316 = Number To Decimal String(number=w3860, width (-)=i16 0) -> (decimal integer string=w3858:string)
                                n2317 = Concatenate Strings(w3858, " s fluorescence event." ("string")) -> (w3856:string)
                                n2318 = local read "Messages"() -> (w3862:string)
                                n2319 = call "Update messages.vi"("Message to add"=w3856, "Old message string"=w3862) -> ("New message string"=w3861:string)
                                n2320 = call <vilib>:"Beep.vi"() -> ()  [unwired: 3 in, 9 out]
                                n2321 = local write "Messages"(w3861) -> ()
                              }
                            }
                            n2322 = node-c288() -> ()  [unwired: 2 out]
                          }
                          n2323 = node-c288(w3837) -> ()  [unwired: 1 out]
                        }
                        frame #2 {
                          n2324 = local write "Fl. High"(FALSE ("Yanking")) -> ()
                        }
                      }
                      n2325 = local read "Trap Delta (MHz)"() -> (w3802:dbl)
                    }
                  }
                }
                frame #1 {
                  n2326 = local read "Stop All"() -> (w3884:bool)
                  n2327 = local read "Fl. Triggered..."() -> (w3882:bool)
                  n2328 = Not(x=w3882) -> (.not. x?=w3883:bool)
                  n2329 = Or(x=w3883, y=w3884) -> (x .or. y?=w3881:bool)
                  n2330 = Not(x=w3881) -> (.not. x?=→"Waiting":bool)
                }
              }
              n2331 = node-c288() -> ()  [unwired: 2 out]
            }
            n2332 = node-c288(w3777) -> ()  [unwired: 1 out]
          }
        }
      }
      event "Stop All": Value Change {
        n2333 = event-data() -> ()  [unwired: 7 out]
        n2334 = local read "Stop All"() -> (w3890:bool)
      }
    }
    n2335 = node-c288() -> ()  [unwired: 2 out]
  }
  n2336 = node-c288(w73) -> ()  [unwired: 1 out]
  n2337 = node-c288(w163) -> ()  [unwired: 1 out]
  n2338 = flat-sequence {
    tunnel: w33 -> [w3895]
    tunnel: [w3894] -> w39
    tunnel: [w3891] -> w38
    tunnel: w37 -> [_]
    tunnel: w36 -> [_]
    tunnel: w35 -> [_]
    tunnel: w34 -> [_]
    tunnel: w32 -> [w3892]
    tunnel: w39 -> [w3898]
    tunnel: w38 -> [w3897]
    frame #0 {
      w3893 = FALSE ("APD to FIFO")
      n2339 = xnode "Read/Write Control"("FPGA VI Reference In"=w3895, "error in"=w3892, "APD to FIFO"=w3893, "AI to FIFO"=w3893) -> ("FPGA VI Reference Out"=w3894:T19, "error out"=w3891:errorcluster)
    }
    frame #1 {
      n2340 = xnode "Invoke Method"("FPGA VI Reference In"=w3898, "error in"=w3897) -> ("FPGA VI Reference Out"=w3896:T19)  [unwired: 1 out]
      n2341 = xnode "Close FPGA VI Reference"("FPGA VI Reference In"=w3896) -> ()  [unwired: 1 in, 1 out]
    }
  }
